vi "draw_blockline.vi"(11 "picture in":picture) -> (3 "picture out":picture)   [LabVIEW 2024]
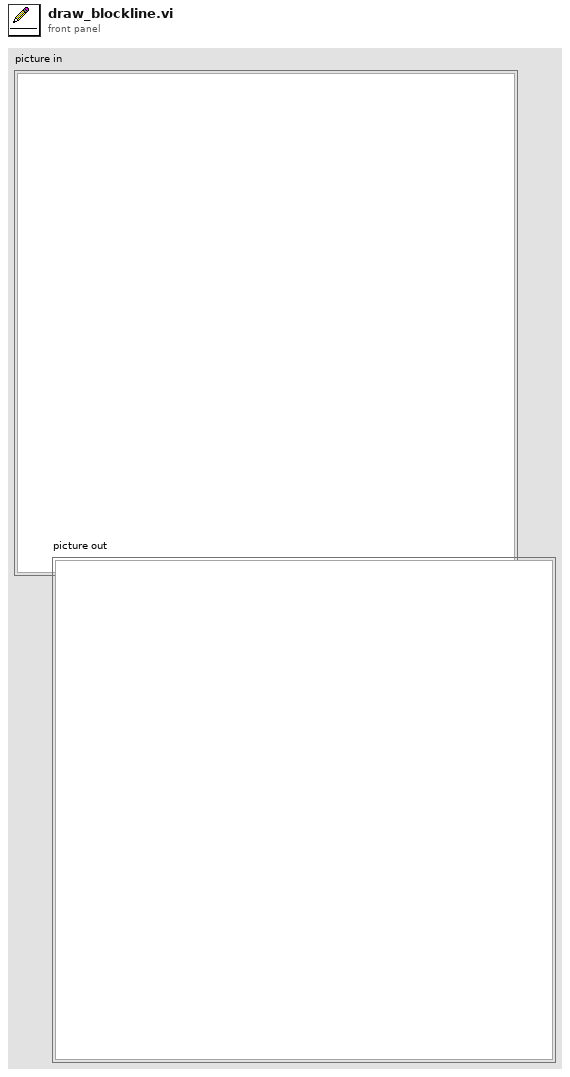
[diagram p1: front panel]
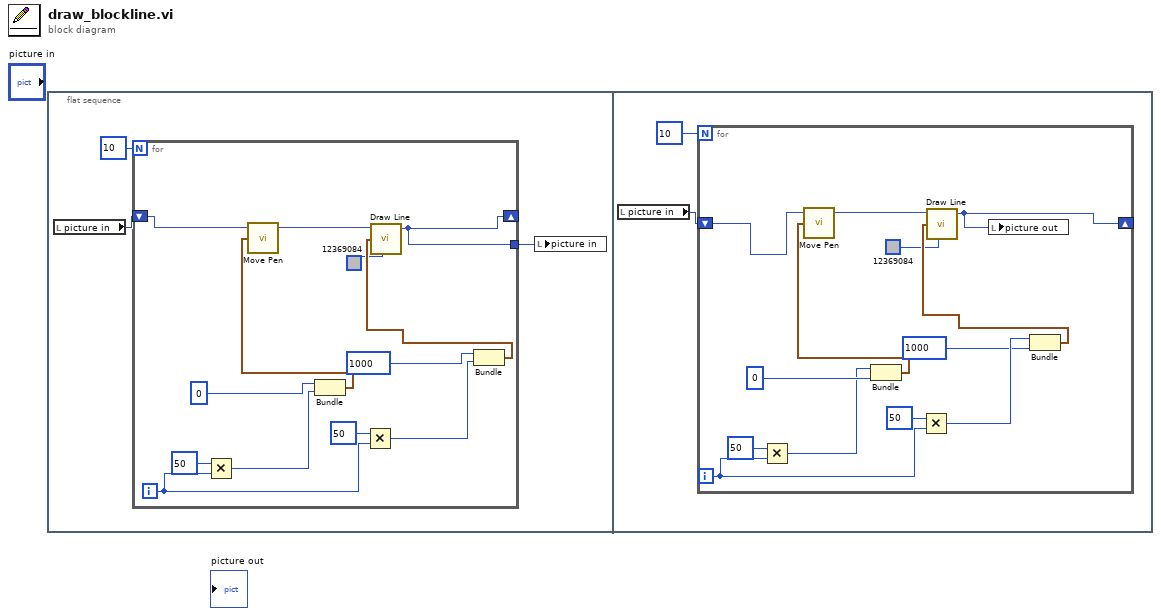
[diagram p0: block diagram]
diagram:
  n1 = flat-sequence {
    frame #0 {
      n2 = local read "picture in"() -> (w1:picture)
      n3 = for {
        N: 10 -> [_]
        tunnel: [w6] -> w2
        shift-right: [w6] -> _
        shift-left: w1 -> [w5]
        i -> [w7]
        n4 = Multiply(x=50, y=w7) -> (x*y=w9:i32)
        n5 = Bundle(0, w9) -> (w14:cluster{i32, i32})  [unwired: 1 in]
        n6 = call <vilib>:"Move Pen.vi"("new position"=w14, "picture"=w5) -> ("new picture"=w13:picture)  [unwired: 3 in]
        n7 = Multiply(x=50, y=w7) -> (x*y=w11:i32)
        n8 = Bundle(1000, w11) -> (w8:cluster{i32, i32})  [unwired: 1 in]
        n9 = call <vilib>:"Draw Line.vi"("picture"=w13, "end point"=w8, "color(black)"=u32 12369084) -> ("new picture"=w6:picture)  [unwired: 6 in]
      }
      n10 = local write "picture in"(w2) -> ()
    }
    frame #1 {
      n11 = local read "picture in"() -> (w17:picture)
      n12 = for {
        N: 10 -> [_]
        shift-right: [w20] -> _
        shift-left: w17 -> [w21]
        i -> [w26]
        n13 = Multiply(x=50, y=w26) -> (x*y=w24:i32)
        n14 = Bundle(w24, 0) -> (w30:cluster{i32, i32})  [unwired: 1 in]
        n15 = call <vilib>:"Move Pen.vi"("new position"=w30, "picture"=w21) -> ("new picture"=w29:picture)  [unwired: 3 in]
        n16 = Multiply(x=50, y=w26) -> (x*y=w23:i32)
        n17 = Bundle(w23, 1000) -> (w27:cluster{i32, i32})  [unwired: 1 in]
        n18 = call <vilib>:"Draw Line.vi"("picture"=w29, "end point"=w27, "color(black)"=u32 12369084) -> ("new picture"=w20:picture)  [unwired: 6 in]
        n19 = local write "picture out"(w20) -> ()
      }
    }
  }
